vi "Ex 06-5 - Multiple Channels B-Scan With Logging.vi"() -> ()   [LabVIEW 2015]
uses:
  <instrlib>/MicroPulse/Public/Data/Datatypes/MP - data formatting.ctl
  <instrlib>/MicroPulse/Public/Data/Datatypes/MP - amplitude reporting mode.ctl
  <instrlib>/MicroPulse/Public/Data/Datatypes/MP - averaging.ctl
  <instrlib>/MicroPulse/Public/Data/Datatypes/MP - transmit parameters.ctl
  <instrlib>/MicroPulse/Public/Data/Datatypes/MP - pulser voltage.ctl
  <instrlib>/MicroPulse/Public/Data/Datatypes/MP - pulse damping.ctl
  <instrlib>/MicroPulse/Public/Data/Datatypes/MP - test parameters.ctl
  <instrlib>/MicroPulse/Public/Data/Datatypes/MP - receive parameters.ctl
  <instrlib>/MicroPulse/Public/Data/Datatypes/MP - display gate.ctl
  <instrlib>/MicroPulse/Public/Data/Datatypes/MP - waveform type.ctl
  <instrlib>/MicroPulse/Public/Data/Datatypes/MP - analogue filter.ctl
  <instrlib>/MicroPulse/Public/Data/Datatypes/MP - frequency filter.ctl
  <instrlib>/MicroPulse/Public/Data/Datatypes/MP - digital filtering.ctl
  <instrlib>/MicroPulse/Public/Data/Datatypes/MP - high pass filter.ctl
  <instrlib>/MicroPulse/Public/Data/Datatypes/MP - low pass filter.ctl
  <instrlib>/MicroPulse/Public/Data/Datatypes/TCP config.ctl
  <instrlib>/MicroPulse/Public/Data/Datatypes/MP - data output format.ctl
  <instrlib>/MicroPulse/Public/Data/Datatypes/MP - sample frequency.ctl
  <instrlib>/MicroPulse/Public/Data/Datatypes/MP - instrument type.ctl
  <instrlib>/MicroPulse/Public/Data/Datatypes/MP - fly scan range (timed).ctl
  <instrlib>/MicroPulse/Public/Data/Datatypes/MP - inspection direction.ctl
  <instrlib>/MicroPulse/Public/Data/Datatypes/PNDT - colour map selector.ctl
  <instrlib>/MicroPulse/Examples/SubVIs/Main Program State - Enum.ctl
  <instrlib>/MicroPulse/Public/Helper VIs/Low Level/FGV - B-Scan Active - Action [Enum].ctl
  <vilib>/ErrorRing/Error Ring.xnode
  <instrlib>/MicroPulse/MicroPulse_Driver.lvlib
panel:
  in  "Colour Map":T1
  out "B-Scan In Progress?":bool
  in  "Stop Scan":bool
  out "live error out":errorcluster
  out "live error out 2":errorcluster
  in  "Centre Cursor 2":bool
  out "B-Scan Chart 2":u16[][](graph)
  in  "Centre Cursor":bool
  out "B-Scan Chart":u16[][](graph)
  out "Instrument Type":T2
  out "Sample Frequency out":T3 caption="Sample Frequency"
  out "Stop":bool
  in  "Sample Frequency":T3
  in  "PRF":u16=20000 caption="[PRF]" min=1 max=20000 step=100 format="%dHz"
  in  "Data Output Format":T4=enum."8-bit Mode" caption="[DOF]"
  out "A-Scan + Peaks 2":cluster{"timebase":dbl[], "data":u16[]}[](graph) caption="A-Scan + Peaks Test 2"
  out "running average PRF 2":dbl format="%0.2f"
  in  "Channel Tab":enum32{"Test 1", "Test 2", "Inspection"}(tab)
  in  "Test 1 Tab":enum32{"Ultrasonic Parameters"}(tab)
  in  "Data Formatting":T5={"Amplitude Mode"=enum."Peaks + Ascan for Multigate", "Averaging"=enum."None", "Coupling Level"=0} {"Coupling Level" max=4095 step=1}
  in  "Transmit Parameters":T8={"Pulse Voltage"=enum."50V", "Pulse Shape"={"Damping"=enum."660W", "Width"=250}} {"Pulse Shape"."Width" min=16 max=1010 step=50 format="%.0fns"}
  in  "Test Parameters":T11={"Test No."=1, "Tx Channel"=1, "Rx Channel"=1} {"Rx Channel" min=1 max=1024; "Tx Channel" min=1 max=1024}
  in  "Receive Parameters":T12={"Display Gate"={"Start"=0.0, "Length"=100.0}, "Delay"=0.0, "Waveform Type"=enum."Rectified Signal", "Gain"=50.0, "Analogue Filtering"={"Bandpass"=enum."No change", "Smoothing"=1}, "Digital Filtering"={"High Pass Filter"=enum."None", "Low Pass Filter"=enum."None"}} {"Delay" format="%#_g us"; "Display Gate"."Length" min=0.0 max=64000.0 step=1.0 format="%#_g us"; "Display Gate"."Start" min=0.0 max=64000.0 step=1.0 format="%#_g us"; "Analogue Filtering"."Smoothing" min=1 max=11 step=1; "Gain" min=-6.0 max=70.0 step=0.25 format="%.2fdB"}
  in  "Test 1 Tab 2":enum32{"Ultrasonic Parameters"}(tab)
  in  "Data Formatting 2":T5={"Amplitude Mode"=enum."Peaks + Ascan for Multigate", "Averaging"=enum."None", "Coupling Level"=0} {"Coupling Level" max=4095 step=1}
  in  "Transmit Parameters 2":T8={"Pulse Voltage"=enum."50V", "Pulse Shape"={"Damping"=enum."660W", "Width"=250}} {"Pulse Shape"."Width" min=16 max=1010 step=50 format="%.0fns"}
  in  "Test Parameters 2":T11={"Test No."=1, "Tx Channel"=2, "Rx Channel"=2} {"Rx Channel" min=1 max=1024; "Tx Channel" min=1 max=1024}
  in  "Receive Parameters 2":T12={"Display Gate"={"Start"=0.0, "Length"=100.0}, "Delay"=0.0, "Waveform Type"=enum."Rectified Signal", "Gain"=50.0, "Analogue Filtering"={"Bandpass"=enum."No change", "Smoothing"=1}, "Digital Filtering"={"High Pass Filter"=enum."None", "Low Pass Filter"=enum."None"}} {"Delay" format="%#_g us"; "Display Gate"."Length" min=0.0 max=64000.0 step=1.0 format="%#_g us"; "Display Gate"."Start" min=0.0 max=64000.0 step=1.0 format="%#_g us"; "Analogue Filtering"."Smoothing" min=1 max=11 step=1; "Gain" min=-6.0 max=70.0 step=0.25 format="%.2fdB"}
  in  "Log Data?":bool caption="Log Data At End Of Scan?"
  out "Scan Timer Enabled?":bool
  in  "Start Timed Test":bool
  in  "Timed Scan definition":T20={"Max Scan Length"=1200, "Update Rate"=500, "Direction"=enum."Forwards"} {"Update Rate" format="%#_6f"; "Max Scan Length" format="%#_6f"}
  out "A-Scan + Peaks":cluster{"timebase":dbl[], "data":u16[]}[](graph) caption="A-Scan + Peaks Test 1"
  in  "Single Scan":bool
  in  "Stop Streaming":bool
  in  "Start Streaming":bool
  out "Command List":string
  in  "QUIT":bool
  out "running average PRF":dbl format="%0.2f"
  out "System Messages":string
  in  "TCP config":T22={"Connection ID"=refnum, "IP address"="10.1.1.2", "host port"=1067, "OC timeout"=5000, "Read timeout"=2000, "Write timeout"=100} {"Write timeout" format="%dms"; "Read timeout" format="%dms"; "OC timeout" format="%dms"}
  # "Example 06-5 - Multiple Channels B-Scan\n\nSet all controls to the required values\nbefore running the VI."
  # "Tx and Rx Channels MUST be set BEFORE running"
  # "TEST 1"
  # "TEST 2"
  # "Set to zero for unlimited points. Requires manual stop."
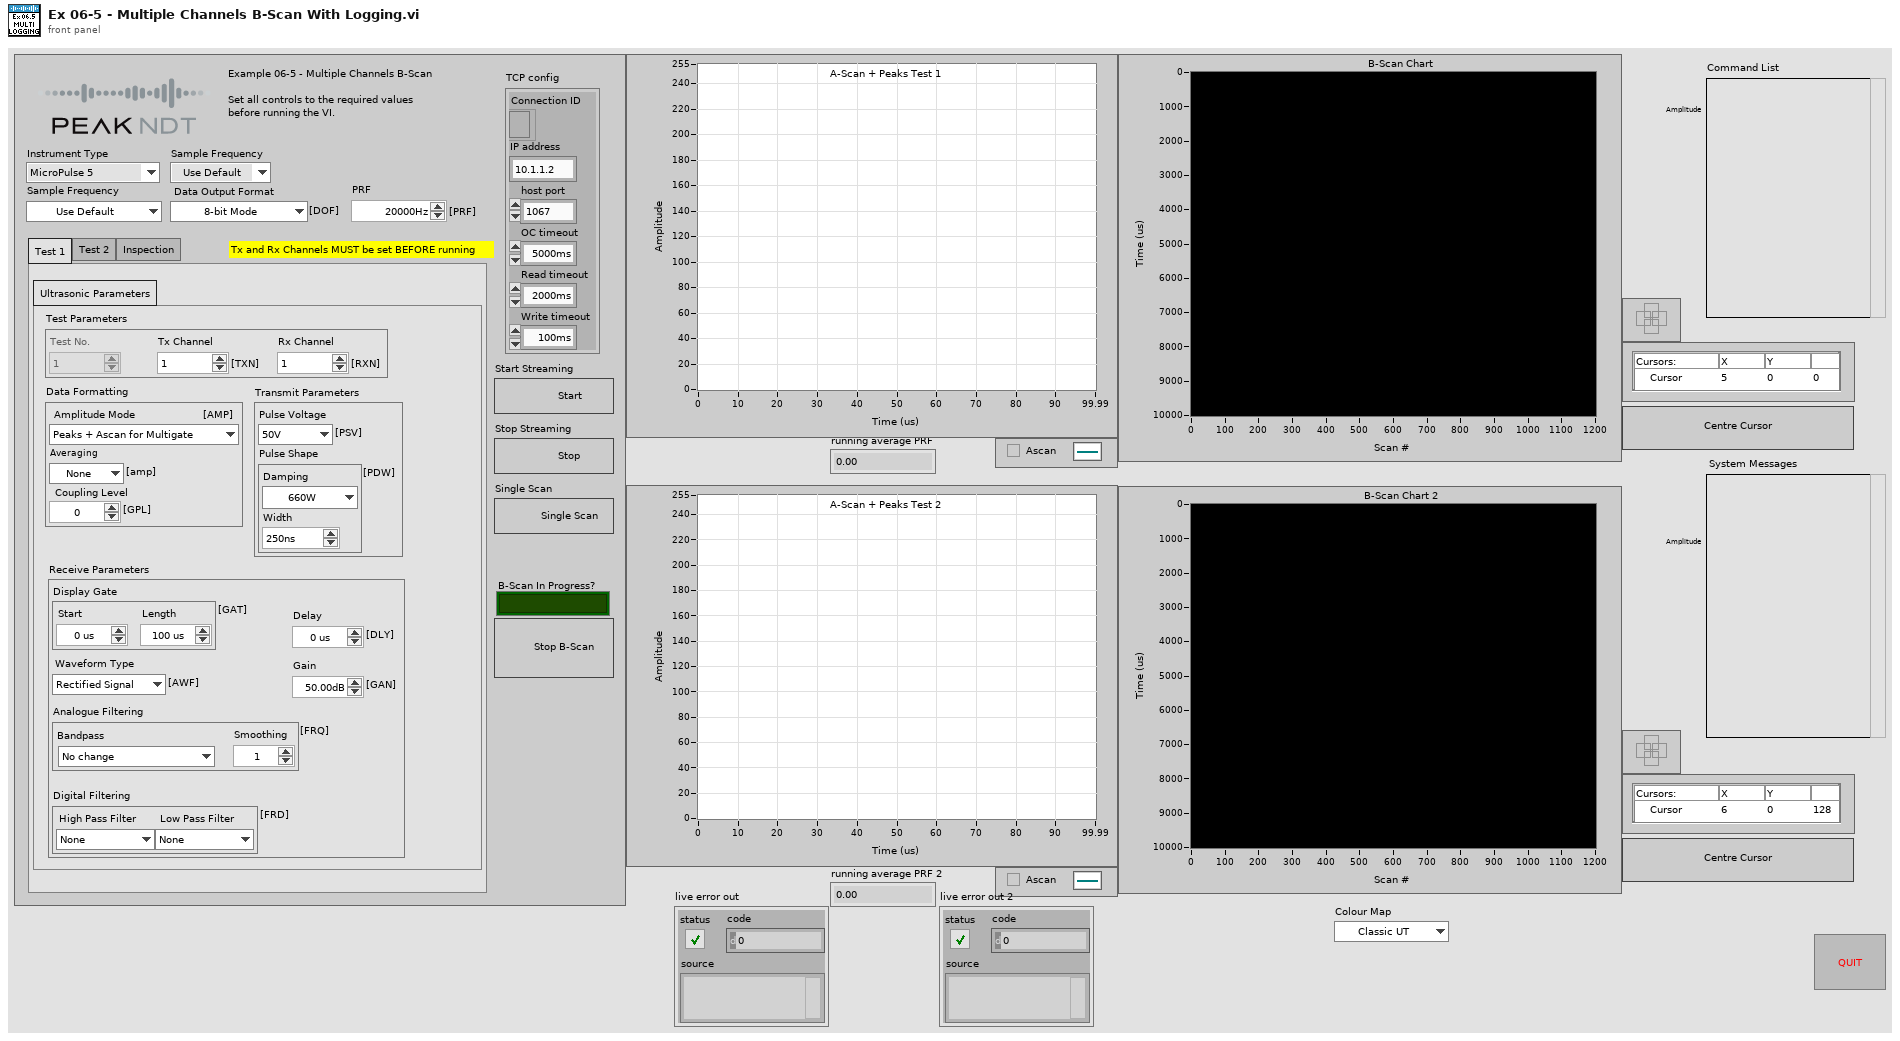
[diagram p1: front panel]
types:
  T1 = typedef "MicroPulse_Driver.lvlib/PNDT - colour map selector.ctl" = enum16{"Classic UT", "Ultrasonic", "Inverse Grey", "Grey Scale", "TOFD", "Fire", "Rainbow", "Ice", "Original"}
  T2 = typedef "MicroPulse_Driver.lvlib/MP - instrument type.ctl" = enum16{"MicroPulse 5", "LT1", "LT2", "LTPA", "MPLT", "MicroPulse 6", "PipeScanner", "<MicroPulse>", "Micropulse 4", "Simulated Data"}
  T3 = typedef "MicroPulse_Driver.lvlib/MP - sample frequency.ctl" = enum16{"Use Default", "200MHz (LT2 only)", "100MHz", "50MHz", "25MHz", "10MHz"}
  T4 = typedef "MicroPulse_Driver.lvlib/MP - data output format.ctl" = enum16{"", "8-bit Mode", "10-bit Mode", "12-bit Mode", "16-bit Mode", "8-bit Log Mode", "12-bit Packed Mode"}
  T5 = typedef "MicroPulse_Driver.lvlib/MP - data formatting.ctl" = cluster{"Amplitude Mode":T6, "Averaging":T7, "Coupling Level":u32}
  T6 = typedef "MicroPulse_Driver.lvlib/MP - amplitude reporting mode.ctl" = enum16{"1st Peak in gate", "Maximum Peak in gate", "All Peaks", "Ascan Data", "1st Threshold Crossing Peak", "Ascan + Peaks", "All Peaks for Multigate", "Peaks + Ascan for Multigate", "Peaks + P_Ascan for Multigate", "Full Matrix Capture"}
  T7 = typedef "MicroPulse_Driver.lvlib/MP - averaging.ctl" = enum16{"None", "2", "4", "8", "16", "32", "64", "128", "256"}
  T8 = typedef "MicroPulse_Driver.lvlib/MP - transmit parameters.ctl" = cluster{"Pulse Voltage":T9, "Pulse Shape":cluster{"Damping":T10, "Width":u32}}
  T9 = typedef "MicroPulse_Driver.lvlib/MP - pulser voltage.ctl" = enum16{"50V", "100V", "150V", "200V", "250V", "300V"}
  T10 = typedef "MicroPulse_Driver.lvlib/MP - pulse damping.ctl" = enum16{"660W", "458W", "220W", "149W", "102W", "82W", "63W", "51W"}
  T11 = typedef "MicroPulse_Driver.lvlib/MP - test parameters.ctl" = cluster{"Test No.":u32, "Tx Channel":u32, "Rx Channel":u32}
  T12 = typedef "MicroPulse_Driver.lvlib/MP - receive parameters.ctl" = cluster{"Display Gate":T13, "Delay":dbl, "Waveform Type":T14, "Gain":dbl, "Analogue Filtering":T15, "Digital Filtering":T17}
  T13 = typedef "MicroPulse_Driver.lvlib/MP - display gate.ctl" = cluster{"Start":dbl, "Length":dbl}
  T14 = typedef "MicroPulse_Driver.lvlib/MP - waveform type.ctl" = enum16{"Rectified Signal", "RF Signal", "+Half Wave", "-Half Wave"}
  T15 = typedef "MicroPulse_Driver.lvlib/MP - analogue filter.ctl" = cluster{"Bandpass":T16, "Smoothing":u16}
  T16 = typedef "MicroPulse_Driver.lvlib/MP - frequency filter.ctl" = enum16{"No change", "1MHz Bandpass", "2MHz Bandpass", "4MHz Bandpass", "5MHz Bandpass", "10MHz Bandpass", "2.5-18MHz Broadband", "0.75-12MHz  Broadband", "0.5MHz Bandpass", "5MHz 2nd Order TOFD", "10MHz 2nd Order TOFD", "3.0-25MHz Broadband", "3.0-30MHz Broadband"}
  T17 = typedef "MicroPulse_Driver.lvlib/MP - digital filtering.ctl" = cluster{"High Pass Filter":T18, "Low Pass Filter":T19}
  T18 = typedef "MicroPulse_Driver.lvlib/MP - high pass filter.ctl" = enum16{"None", "0.7MHz", "1.5MHz", "4.0MHz", "7.5MHz", "10.0MHz", "User Defined"}
  T19 = typedef "MicroPulse_Driver.lvlib/MP - low pass filter.ctl" = enum16{"None", "1.8MHz", "3.0MHz", "6.0MHz", "8.0MHz", "12.0MHz", "User Defined"}
  T20 = typedef "MicroPulse_Driver.lvlib/MP - fly scan range (timed).ctl" = cluster{"Max Scan Length":i32, "Update Rate":i32, "Direction":T21}
  T21 = typedef "MicroPulse_Driver.lvlib/MP - inspection direction.ctl" = enum16{"Forwards", "Backwards"}
  T22 = typedef "MicroPulse_Driver.lvlib/TCP config.ctl" = cluster{"Connection ID":refnum<k5>, "IP address":string, "host port":u16, "OC timeout":i32, "Read timeout":i32, "Write timeout":i32}
  T23 = typedef "Main Program State - Enum.ctl" = enum16{"Initialise", "Init HW", "Run", "Reset HW", "Shutdown"}
  T24 = typedef "MicroPulse_Driver.lvlib/FGV - B-Scan Active - Action [Enum].ctl" = enum16{"Read", "Read & Reset Start Flag", "Start B-Scan", "B-Scan Finished"}
  T25 = typedef "MicroPulse_Driver.lvlib/MP-Registry Data-Cluster.ctl" = cluster{"Instrument Type":T2, "Serial #":u64, "Sample Frequency":T3, "dt (us)":dbl, "DOF":T4, "Material Velocity":dbl, "Asynch Reads":T26, "NUM of Tests":u32, "System Details":T27, "Gates":T29[], "Encoders":T35[], "CMD LUT":variant, "Command List":string}
  T26 = typedef "MicroPulse_Driver.lvlib/MP - asynch read mode.ctl" = enum16{"Disabled", "Enabled"}
  T27 = typedef "MicroPulse_Driver.lvlib/MP - general system status.ctl" = cluster{"System Type":T2, "Serial No.":u64, "Channels":cluster{"Conv":u8, "PA":u16, "Extra":u32}, "Sample Frequency":cluster{"Default":u8, "Actual":u8}, "Software Versions":string, "Data Output Format":cluster{"Default":T4, "Actual":T4}, "Temperatures":cluster{"System":u8, "Processor":u8, "Slave Sys":u8, "Slave Proc":u8}, "Tx Buffer Size":u32, "System Error":string, "No. of Cards":u8, "DAC Gain":i16, "Uptimes":cluster{"since Power":u32, "since RSTS":u32, "since SRST":u32}, "Voltages":cluster{"Nominal":dbl, "Measured":dbl, "Difference":dbl}[], "Interface Cards":T28[]}
  T28 = typedef "MicroPulse_Driver.lvlib/MP - interface card status.ctl" = cluster{"Status":u8, "Map":u8, "Board - T":u8, "FPGA - T":u8, "PAIF Status":string, "Version":string}
  T29 = typedef "MicroPulse_Driver.lvlib/MP - Registry Gates.ctl" = cluster{"Display Gate":T13, "ETM Mode":T30, "Echo Gate":T31, "Insp Gates":T32[]}
  T30 = typedef "MicroPulse_Driver.lvlib/MP - echo gate mode.ctl" = enum16{"Echo Trigger OFF", "Echo Gate Display Mode", "Echo Trigger ON", "Multi Gate or FMC Mode", "Reserved", "PA - Echo Trigger ON"}
  T31 = typedef "MicroPulse_Driver.lvlib/MP - echo gate parameters.ctl" = cluster{"Start (us)":dbl, "Length (us)":dbl, "Threshold":u16, "Colour":u32}
  T32 = typedef "MicroPulse_Driver.lvlib/MP - multigate inspection gate parameters.ctl" = cluster{"Start (us)":dbl, "Length (us)":dbl, "Threshold":u16, "Enabled?":bool, "Max # Peaks":u16, "Hysteresis":T33, "Mode":T34, "Inverted?":bool, "Colour ":u32}
  T33 = typedef "MicroPulse_Driver.lvlib/MP - hysteresis level.ctl" = enum16{"None", "3dB", "6dB", "9dB", "12dB"}
  T34 = typedef "MicroPulse_Driver.lvlib/MP - multigate mode.ctl" = enum16{"1st Peak in Gate", "Largest Peak In Gate", "All Peaks In Gate", "1st Threshold Crossing"}
  T35 = typedef "MicroPulse_Driver.lvlib/MP - encoder settings.ctl" = cluster{"Encoder Type":T36, "Counts/mm":u32, "Enable Termination?":bool, "Multiplier":u32, "Backlash Period (s)":dbl, "Encoder Filter":u32}
  T36 = typedef "MicroPulse_Driver.lvlib/MP - encoder type.ctl" = enum16{"Quadrature", "Step/Direction"}
  T37 = typedef "MicroPulse_Driver.lvlib/MP - scan data info.ctl" = cluster{"Message Header":u16, "Error Message":u16, "Test No.":u32, "Channel No.":u8, "Sweep No.":u32, "Gate No.":u32, "DOF":T4, "retain data":T38, "scan data":u16[], "scan length":i32, "scan index":i32, "peak data":cluster{"timebase":u16[], "data":u16[]}, "#peaks":i32, "PRF":dbl, "IP":cluster{"Axis No.":u8, "Location":u32, "MIP location":u32, "MIP?":bool}, "echo range":u16, "ETG":bool, "CAL 0 complete":bool, "Axis Positions":T39}
  T38 = typedef "MicroPulse_Driver.lvlib/MP - retain scan.ctl" = enum16{"None", "Ascan", "Peaks"}
  T39 = typedef "MicroPulse_Driver.lvlib/MP - axis positions (LLC).ctl" = cluster{"Axis 1":u32, "Axis 2":u32, "Axis 3":u32, "Axis 4":u32, "Status":u8}
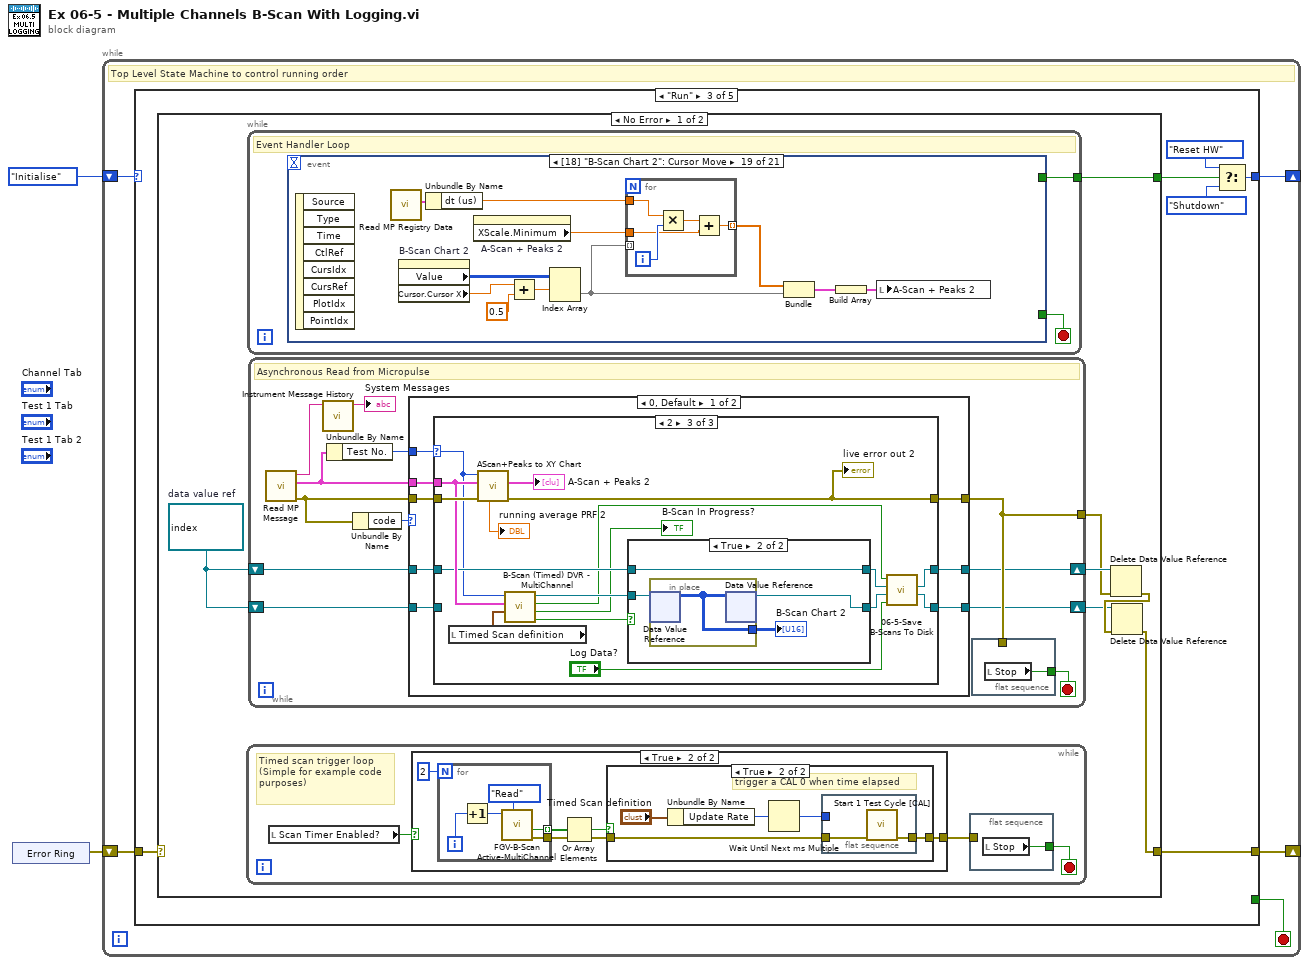
[diagram p0: block diagram]
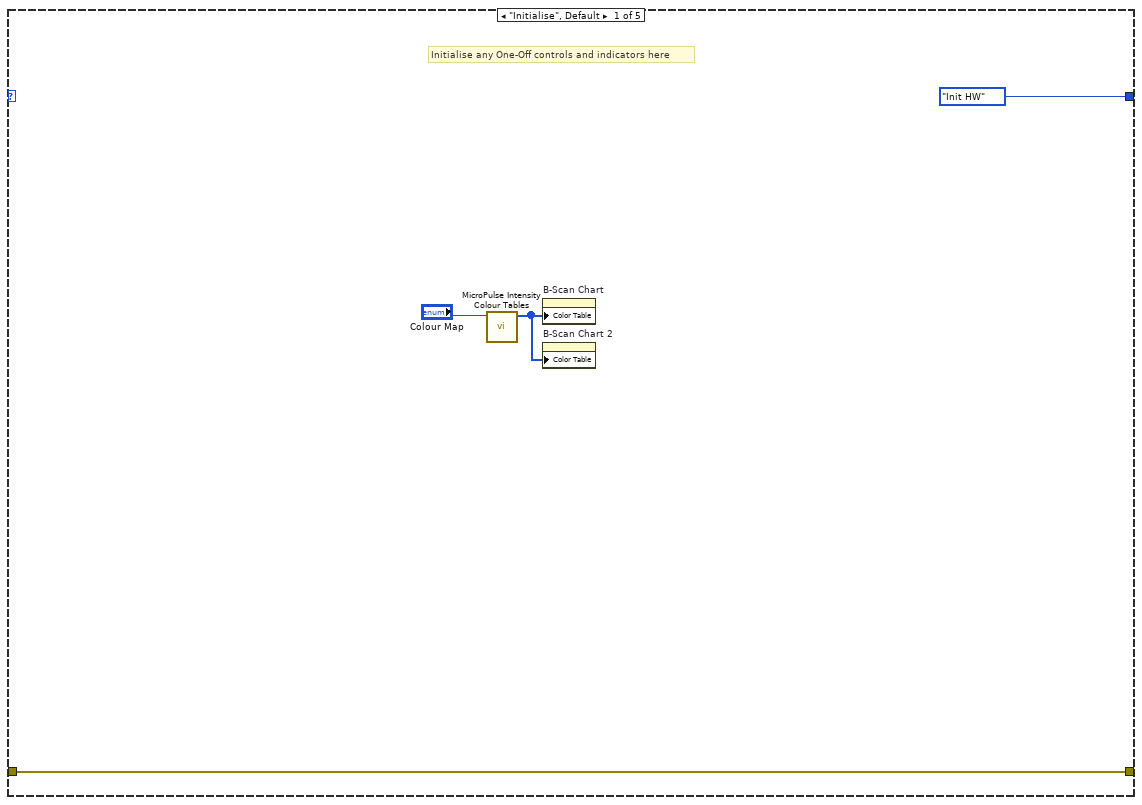
[diagram p2: hidden frame]
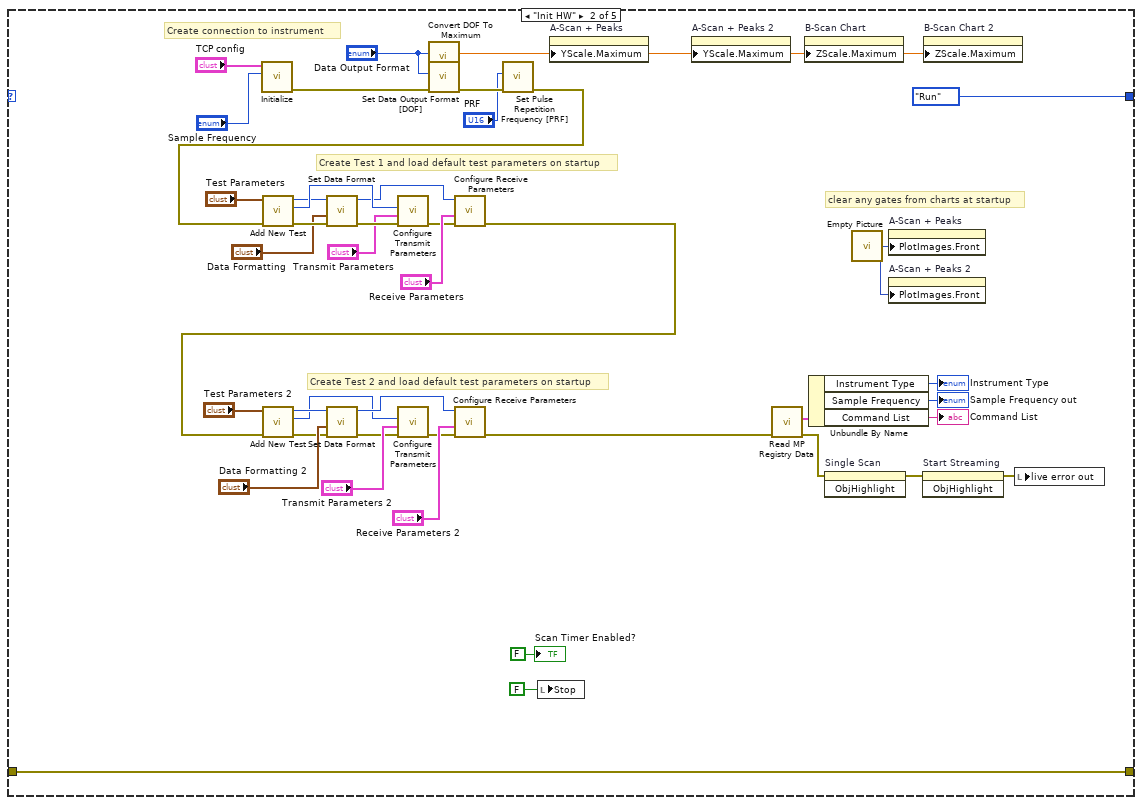
[diagram p3: hidden frame]
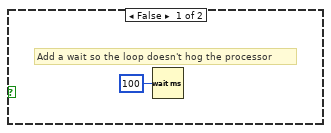
[diagram p4: hidden frame]
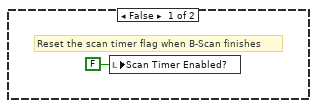
[diagram p5: hidden frame]
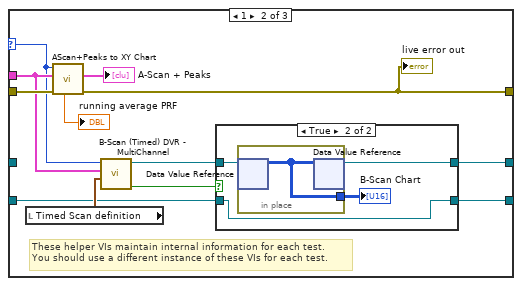
[diagram p7: hidden frame]
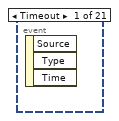
[diagram p11: hidden frame]
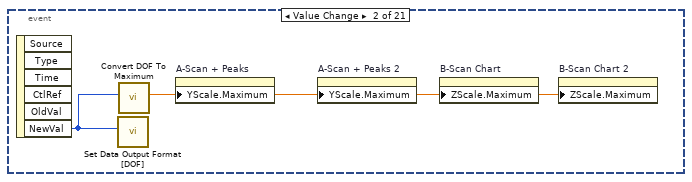
[diagram p12: hidden frame]
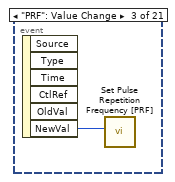
[diagram p13: hidden frame]
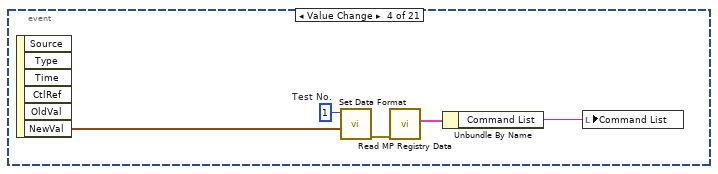
[diagram p14: hidden frame]
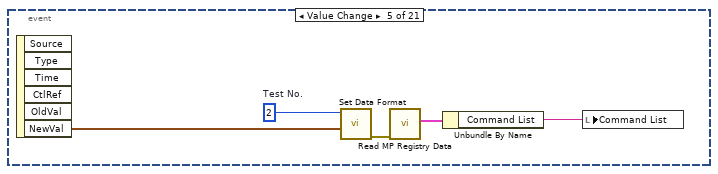
[diagram p15: hidden frame]
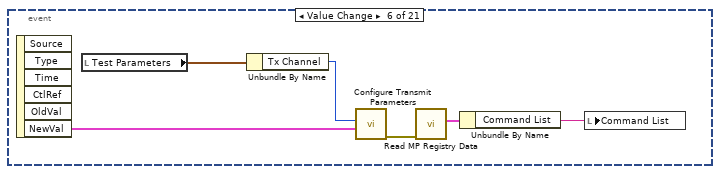
[diagram p16: hidden frame]
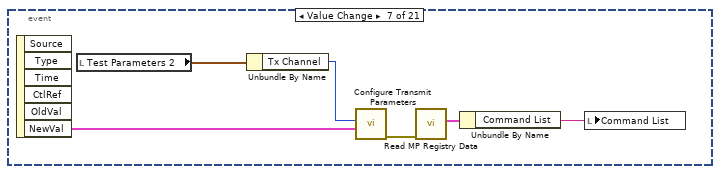
[diagram p17: hidden frame]
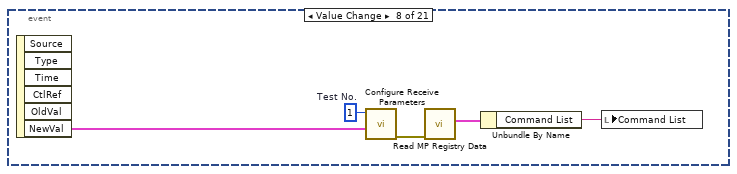
[diagram p18: hidden frame]
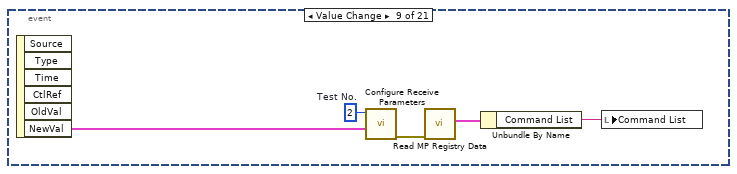
[diagram p19: hidden frame]
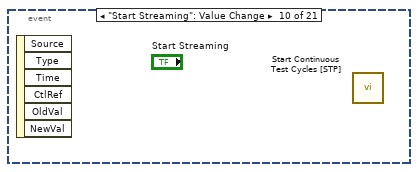
[diagram p20: hidden frame]
diagram:
  n1 = xnode "Error Ring"() -> ("error out"=w2:errorcluster)
  n2 = while {
    shift-right: [w4] -> _
    shift-left: Main_Program_State_-_Enum."Initialise" -> [w7]
    shift-right: [w5] -> _
    shift-left: w2 -> [w6]
    stop <- w3 stop-if-true
    # "Top Level State Machine to control running order"
    n3 = case shown="\"Run\"" w7 {
      tunnel: w6 -> [w10 w28 w59 w276 w281]
      tunnel: [w10 w28 w58 w275 w281] -> w5
      tunnel: [Main_Program_State_-_Enum."Init HW" Main_Program_State_-_Enum."Run" w54 Main_Program_State_-_Enum."Init HW" Main_Program_State_-_Enum."Initialise"] -> w4
      tunnel: [_ _ _ _ TRUE] -> w3
      frame "Initialise", Default {
        # "Initialise any One-Off controls and indicators here"
        n4 = call <instrlib>:"MicroPulse Intensity Colour Tables.vi"("Colour Map Type"="Colour Map") -> ("Colour Table"=w8:u32[])  [unwired: 10 in]
        n5 = property on="B-Scan Chart" class="IntGraph (strict)"("Color Table"=w8) -> ()  [unwired: 2 in, 2 out]
        n6 = property on="B-Scan Chart 2" class="IntGraph (strict)"("Color Table"=w8) -> ()  [unwired: 2 in, 2 out]
      }
      frame "Init HW" {
        # "Create connection to instrument"
        # "Create Test 2 and load default test parameters on startup"
        # "clear any gates from charts at startup"
        # "Create Test 1 and load default test parameters on startup"
        n7 = call <instrlib>:"Initialize.vi"("Sample Frequency"="Sample Frequency", "TCP config"="TCP config") -> ("error out"=w21:errorcluster)  [unwired: 8 in, 1 out]
        n8 = call <instrlib>:"Convert DOF To Maximum.vi"("Data Output Format"="Data Output Format") -> ("Data Maximum"=w12:dbl)  [unwired: 10 in]
        n9 = call <instrlib>:"Set Data Output Format [DOF].vi"("error in (no error)"=w21, "Mode"="Data Output Format") -> ("error out"=w23:errorcluster)  [unwired: 8 in, 1 out]
        n10 = call <instrlib>:"Set Pulse Repetition Frequency [PRF].vi"("error in (no error)"=w23, "Frequency (Hz)"="PRF") -> ("error out"=w20:errorcluster)  [unwired: 8 in, 1 out]
        n11 = call <instrlib>:"Add New Test.vi"("error in (no error)"=w20, "Test Parameters"="Test Parameters") -> ("error out"=w39:errorcluster, "Tx Channel out"=w38:u32, "Test No. out"=w36:u32)  [unwired: 6 in, 1 out]
        n12 = call <instrlib>:"Set Data Format.vi"("error in (no error)"=w39, "Data Formatting"="Data Formatting", "Test No."=w36) -> ("error out"=w33:errorcluster, "Test No. out"=w37:u32)  [unwired: 6 in, 1 out]
        n13 = call <instrlib>:"Configure Transmit Parameters.vi"("error in (no error)"=w33, "Transmit Parameters"="Transmit Parameters", "Tx Channel"=w38) -> ("error out"=w32:errorcluster)  [unwired: 7 in, 1 out]
        n14 = call <instrlib>:"Configure Receive Parameters.vi"("error in (no error)"=w32, "Receive Parameters"="Receive Parameters", "Test No."=w37) -> ("error out"=w16:errorcluster)  [unwired: 6 in, 2 out]
        n15 = call <instrlib>:"Add New Test.vi"("error in (no error)"=w16, "Test Parameters"="Test Parameters 2") -> ("error out"=w48:errorcluster, "Tx Channel out"=w44:u32, "Test No. out"=w46:u32)  [unwired: 6 in, 1 out]
        n16 = call <instrlib>:"Set Data Format.vi"("error in (no error)"=w48, "Data Formatting"="Data Formatting 2", "Test No."=w46) -> ("error out"=w49:errorcluster, "Test No. out"=w45:u32)  [unwired: 6 in, 1 out]
        n17 = call <instrlib>:"Configure Transmit Parameters.vi"("error in (no error)"=w49, "Transmit Parameters"="Transmit Parameters 2", "Tx Channel"=w44) -> ("error out"=w50:errorcluster)  [unwired: 7 in, 1 out]
        n18 = call <instrlib>:"Configure Receive Parameters.vi"("error in (no error)"=w50, "Receive Parameters"="Receive Parameters 2", "Test No."=w45) -> ("error out"=w15:errorcluster)  [unwired: 6 in, 2 out]
        n19 = local write "Stop"(FALSE ("stop")) -> ()
        n20 = property on="A-Scan + Peaks" class="XYGraph (strict)"("YScale.Maximum"=w12) -> ()  [unwired: 2 in, 2 out]
        n21 = property on="A-Scan + Peaks 2" class="XYGraph (strict)"("YScale.Maximum"=w12) -> ()  [unwired: 2 in, 2 out]
        n22 = call <instrlib>:"Read MP Registry Data.vi"("error in (no error)"=w15) -> ("error out"=w42:errorcluster, "Micropulse Data"=w40:T25)  [unwired: 7 in, 2 out]
        n23 = property on="B-Scan Chart" class="IntGraph (strict)"("ZScale.Maximum"=w12) -> ()  [unwired: 2 in, 2 out]
        n24 = Unbundle By Name(w40) -> ("Instrument Type"=→"Instrument Type":T2, "Sample Frequency"=→"Sample Frequency out":T3, "Command List"=→"Command List":string)
        n25 = invoke on="Single Scan" class="Bool" method="ObjHighlight"(error in=w42) -> (error out=w43:errorcluster)  [unwired: 2 in, 2 out]
        n26 = call "Empty Picture"() -> ("empty picture"=w27:picture)
        n27 = property on="A-Scan + Peaks" class="XYGraph (strict)"("PlotImages.Front"=w27) -> ()  [unwired: 2 in, 2 out]
        n28 = property on="A-Scan + Peaks 2" class="XYGraph (strict)"("PlotImages.Front"=w27) -> ()  [unwired: 2 in, 2 out]
        n29 = invoke on="Start Streaming" class="Bool" method="ObjHighlight"(error in=w43) -> (error out=w13:errorcluster)  [unwired: 2 in, 2 out]
        n30 = property on="B-Scan Chart 2" class="IntGraph (strict)"("ZScale.Maximum"=w12) -> ()  [unwired: 2 in, 2 out]
        n31 = local write "live error out"(w13) -> ()
        "Scan Timer Enabled?" <- FALSE ("Scan Timer Enabled?")
      }
      frame "Run" {
        n32 = case shown="No Error" w59 {
          selector: w59 -> [_ w274]
          tunnel: [w61 w274] -> w58
          tunnel: [w66 _] -> w55
          frame No Error {
            w65 = refnum<data-value> refnum  # data value ref
            n33 = while {
              stop <- w68 stop-if-true
              # "Timed scan trigger loop\n(Simple for example code purposes)"
              n34 = local read "Scan Timer Enabled?"() -> (w69:bool)
              n35 = case shown="True" w69 {
                tunnel: [_ w72] -> w67
                frame False {
                  # "Add a wait so the loop doesn't hog the processor"
                  n36 = Wait (ms)(milliseconds to wait=u32 100) -> ()  [unwired: 1 out]
                }
                frame True {
                  n37 = for {
                    N: 2 -> [_]
                    tunnel: [w80] -> w76 mode=indexing
                    tunnel: [w79] -> w75
                    i -> [w77]
                    n38 = Increment(x=w77) -> (x+1=w78:i32)
                    n39 = call <instrlib>:"FGV-B-Scan Active-MultiChannel.vi"("Action"=FGV_-_B-Scan_Active_-_Action_[Enum]."Read", "Test #"=w78) -> ("error out"=w79:errorcluster, "B-Scan In Progress?"=w80:bool)  [unwired: 7 in, 1 out]
                  }
                  n40 = Or Array Elements(Boolean array=w76) -> (logical OR=w73:bool)
                  n41 = case shown="True" w73 {
                    tunnel: w75 -> [_ w85]
                    tunnel: [_ w83] -> w72
                    frame False {
                      # "Reset the scan timer flag when B-Scan finishes"
                      n42 = local write "Scan Timer Enabled?"(FALSE ("Scan Timer Enabled?")) -> ()
                    }
                    frame True {
                      # "trigger a CAL 0 when time elapsed"
                      n43 = Unbundle By Name("Timed Scan definition") -> ("Update Rate"=w87:i32)
                      n44 = Wait Until Next ms Multiple(millisecond multiple=w87) -> (millisecond timer value=w86:u32)
                      n45 = flat-sequence {
                        tunnel: w86 -> [_]
                        tunnel: w85 -> [w89]
                        tunnel: [w88] -> w83
                        frame #0 {
                          n46 = call <instrlib>:"Start 1 Test Cycle [CAL].vi"("error in (no error)"=w89) -> ("error out"=w88:errorcluster)  [unwired: 9 in, 1 out]
                        }
                      }
                    }
                  }
                }
              }
              n47 = flat-sequence {
                tunnel: [w70] -> w68
                tunnel: w67 -> [_]
                frame #0 {
                  n48 = local read "Stop"() -> (w70:bool)
                }
              }
            }
            n49 = while {
              tunnel: [w160] -> w66
              stop <- w161 stop-if-true
              # "Event Handler Loop"
              n50 = event shown="[18] \"B-Scan Chart 2\": Cursor Move" {
                selector: _ -> [_ _ _ _ _ _ _ _ _ _ _ _ _ _ _ _ _ _ _ _ _]
                dyn-events: _ -> [_ _ _ _ _ _ _ _ _ _ _ _ _ _ _ _ _ _ _ _ _]
                timeout: _ -> [_ _ _ _ _ _ _ _ _ _ _ _ _ _ _ _ _ _ _ _ _]
                tunnel: [_ _ _ _ _ _ _ _ _ _ _ _ w198 _ _ _ _ _ _ _ TRUE ("stop")] -> w161
                tunnel: [_ _ _ _ _ _ _ _ _ _ _ _ TRUE _ _ _ _ _ _ _ _] -> w160
                event Timeout {
                  n51 = event-data() -> ()  [unwired: 1 in, 3 out]
                }
                event Value Change {
                  n52 = event-data() -> ("NewVal"=w163:T4)  [unwired: 1 in, 5 out]
                  n53 = call <instrlib>:"Set Data Output Format [DOF].vi"("Mode"=w163) -> ()  [unwired: 9 in, 2 out]
                  n54 = call <instrlib>:"Convert DOF To Maximum.vi"("Data Output Format"=w163) -> ("Data Maximum"=w162:dbl)  [unwired: 10 in]
                  n55 = property on="A-Scan + Peaks" class="XYGraph (strict)"("YScale.Maximum"=w162) -> ()  [unwired: 2 in, 2 out]
                  n56 = property on="A-Scan + Peaks 2" class="XYGraph (strict)"("YScale.Maximum"=w162) -> ()  [unwired: 2 in, 2 out]
                  n57 = property on="B-Scan Chart" class="IntGraph (strict)"("ZScale.Maximum"=w162) -> ()  [unwired: 2 in, 2 out]
                  n58 = property on="B-Scan Chart 2" class="IntGraph (strict)"("ZScale.Maximum"=w162) -> ()  [unwired: 2 in, 2 out]
                }
                event "PRF": Value Change {
                  n59 = event-data() -> ("NewVal"=w164:u16)  [unwired: 1 in, 5 out]
                  n60 = call <instrlib>:"Set Pulse Repetition Frequency [PRF].vi"("Frequency (Hz)"=w164) -> ()  [unwired: 9 in, 2 out]
                }
                event Value Change {
                  w166 = u32 1  # Test No.
                  n61 = event-data() -> ("NewVal"=w165:T5)  [unwired: 1 in, 5 out]
                  n62 = call <instrlib>:"Set Data Format.vi"("Data Formatting"=w165, "Test No."=w166) -> ("error out"=w169:errorcluster)  [unwired: 7 in, 2 out]
                  n63 = call <instrlib>:"Read MP Registry Data.vi"("error in (no error)"=w169) -> ("Micropulse Data"=w168:T25)  [unwired: 7 in, 3 out]
                  n64 = Unbundle By Name(w168) -> ("Command List"=w167:string)
                  n65 = local write "Command List"(w167) -> ()
                }
                event Value Change {
                  w171 = u32 2  # Test No.
                  n66 = event-data() -> ("NewVal"=w170:T5)  [unwired: 1 in, 5 out]
                  n67 = call <instrlib>:"Set Data Format.vi"("Data Formatting"=w170, "Test No."=w171) -> ("error out"=w174:errorcluster)  [unwired: 7 in, 2 out]
                  n68 = call <instrlib>:"Read MP Registry Data.vi"("error in (no error)"=w174) -> ("Micropulse Data"=w173:T25)  [unwired: 7 in, 3 out]
                  n69 = Unbundle By Name(w173) -> ("Command List"=w172:string)
                  n70 = local write "Command List"(w172) -> ()
                }
                event Value Change {
                  n71 = event-data() -> ("NewVal"=w179:T8)  [unwired: 1 in, 5 out]
                  n72 = local read "Test Parameters"() -> (w180:T11)
                  n73 = Unbundle By Name(w180) -> ("Tx Channel"=w178:u32)
                  n74 = call <instrlib>:"Configure Transmit Parameters.vi"("Transmit Parameters"=w179, "Tx Channel"=w178) -> ("error out"=w176:errorcluster)  [unwired: 8 in, 1 out]
                  n75 = call <instrlib>:"Read MP Registry Data.vi"("error in (no error)"=w176) -> ("Micropulse Data"=w177:T25)  [unwired: 7 in, 3 out]
                  n76 = Unbundle By Name(w177) -> ("Command List"=w175:string)
                  n77 = local write "Command List"(w175) -> ()
                }
                event Value Change {
                  n78 = event-data() -> ("NewVal"=w185:T8)  [unwired: 1 in, 5 out]
                  n79 = local read "Test Parameters 2"() -> (w186:T11)
                  n80 = Unbundle By Name(w186) -> ("Tx Channel"=w184:u32)
                  n81 = call <instrlib>:"Configure Transmit Parameters.vi"("Transmit Parameters"=w185, "Tx Channel"=w184) -> ("error out"=w182:errorcluster)  [unwired: 8 in, 1 out]
                  n82 = call <instrlib>:"Read MP Registry Data.vi"("error in (no error)"=w182) -> ("Micropulse Data"=w183:T25)  [unwired: 7 in, 3 out]
                  n83 = Unbundle By Name(w183) -> ("Command List"=w181:string)
                  n84 = local write "Command List"(w181) -> ()
                }
                event Value Change {
                  w187 = u32 1  # Test No.
                  n85 = event-data() -> ("NewVal"=w191:T12)  [unwired: 1 in, 5 out]
                  n86 = call <instrlib>:"Configure Receive Parameters.vi"("Receive Parameters"=w191, "Test No."=w187) -> ("error out"=w190:errorcluster)  [unwired: 7 in, 2 out]
                  n87 = call <instrlib>:"Read MP Registry Data.vi"("error in (no error)"=w190) -> ("Micropulse Data"=w188:T25)  [unwired: 7 in, 3 out]
                  n88 = Unbundle By Name(w188) -> ("Command List"=w189:string)
                  n89 = local write "Command List"(w189) -> ()
                }
                event Value Change {
                  w192 = u32 2  # Test No.
                  n90 = event-data() -> ("NewVal"=w196:T12)  [unwired: 1 in, 5 out]
                  n91 = call <instrlib>:"Configure Receive Parameters.vi"("Receive Parameters"=w196, "Test No."=w192) -> ("error out"=w195:errorcluster)  [unwired: 7 in, 2 out]
                  n92 = call <instrlib>:"Read MP Registry Data.vi"("error in (no error)"=w195) -> ("Micropulse Data"=w193:T25)  [unwired: 7 in, 3 out]
                  n93 = Unbundle By Name(w193) -> ("Command List"=w194:string)
                  n94 = local write "Command List"(w194) -> ()
                }
                event "Start Streaming": Value Change {
                  n95 = event-data() -> ()  [unwired: 1 in, 6 out]
                  n96 = call <instrlib>:"Start Continuous Test Cycles [STP].vi"() -> ()  [unwired: 10 in, 2 out]
                }
                event "Stop Streaming": Value Change {
                  w197 = TRUE  # Erase All? (def F)
                  n97 = event-data() -> ()  [unwired: 1 in, 6 out]
                  n98 = call <instrlib>:"Enter Idle Mode [STX].vi"("Erase All? (def T)"=w197) -> ()  [unwired: 9 in, 2 out]
                }
                event "Single Scan": Value Change {
                  n99 = event-data() -> ()  [unwired: 1 in, 6 out]
                  n100 = call <instrlib>:"Start 1 Test Cycle [CAL].vi"() -> ()  [unwired: 10 in, 2 out]
                }
                event Value Change {
                  w198 = TRUE
                  # "Stop all activity and reset the hardware to change the sampling frequency"
                  n101 = event-data() -> ()  [unwired: 1 in, 6 out]
                  n102 = local write "Stop"(w198) -> ()
                }
                event "Start Timed Test": Value Change {
                  # "use property node so we can sequence starting\nthe B-Scan acitve flags and then enabling the timer"
                  # "Stop any acquisition that's going on"
                  n103 = event-data() -> ()  [unwired: 1 in, 6 out]
                  n104 = call <instrlib>:"Enter Idle Mode [STX].vi"() -> ("error out"=w203:errorcluster)  [unwired: 10 in, 1 out]
                  n105 = for {
                    N: 2 -> [_]
                    tunnel: FGV_-_B-Scan_Active_-_Action_[Enum]."Start B-Scan" ("Action") -> [w209]
                    shift-right: [w207] -> w202
                    shift-left: w203 -> [w208]
                    i -> [w205]
                    n106 = Increment(x=w205) -> (x+1=w206:i32)
                    n107 = call <instrlib>:"FGV-B-Scan Active-MultiChannel.vi"("Action"=w209, "error in (no error)"=w208, "Test #"=w206) -> ("error out"=w207:errorcluster)  [unwired: 6 in, 2 out]
                  }
                  n108 = property on="Scan Timer Enabled?" class="Bool (strict)"(error in=w202, "Value"=TRUE ("Scan Timer Enabled?")) -> ()  [unwired: 1 in, 2 out]
                }
                event "Stop Scan": Value Change {
                  n109 = event-data() -> ()  [unwired: 1 in, 6 out]
                  n110 = for {
                    N: 2 -> [_]
                    tunnel: [w216] -> w212 mode=indexing
                    tunnel: [w215] -> _
                    i -> [w213]
                    n111 = Increment(x=w213) -> (x+1=w214:i32)
                    n112 = call <instrlib>:"FGV-B-Scan Active-MultiChannel.vi"("Action"=FGV_-_B-Scan_Active_-_Action_[Enum]."Read", "Test #"=w214) -> ("error out"=w215:errorcluster, "B-Scan In Progress?"=w216:bool)  [unwired: 7 in, 1 out]
                  }
                  n113 = Or Array Elements(Boolean array=w212) -> (logical OR=w210:bool)
                  n114 = case shown="True" w210 {
                    frame False {
                    }
                    frame True {
                      n115 = call <instrlib>:"Enter Idle Mode [STX].vi"("Erase All? (def T)"=FALSE) -> ("error out"=w220:errorcluster)  [unwired: 9 in, 1 out]
                      n116 = for {
                        N: 2 -> [_]
                        tunnel: FGV_-_B-Scan_Active_-_Action_[Enum]."B-Scan Finished" ("Action") -> [w225]
                        tunnel: w220 -> [w224]
                        i -> [w223]
                        n117 = Increment(x=w223) -> (x+1=w222:i32)
                        n118 = call <instrlib>:"FGV-B-Scan Active-MultiChannel.vi"("Action"=w225, "error in (no error)"=w224, "Test #"=w222) -> ()  [unwired: 6 in, 3 out]
                      }
                    }
                  }
                }
                event "Centre Cursor": Value Change {
                  n119 = event-data() -> ()  [unwired: 1 in, 6 out]
                  n120 = property on="B-Scan Chart" class="IntGraph (strict)"() -> ("XScale.Maximum"=w231:dbl, "XScale.Minimum"=w227:dbl)  [unwired: 2 in, 2 out]
                  n121 = Subtract(x=w231, y=w227) -> (x-y=w230:dbl)
                  n122 = Divide(x=w230, y=2.0) -> (x/y=w228:dbl)
                  n123 = Add(x=w228, y=w227) -> (x+y=w226:dbl)
                  n124 = property on="B-Scan Chart" class="IntGraph (strict)"("Cursor.Cursor X"=w226) -> ()  [unwired: 2 in, 2 out]
                }
                event "B-Scan Chart": Cursor Move {
                  n125 = event-data() -> ()  [unwired: 1 in, 8 out]
                  n126 = call <instrlib>:"Read MP Registry Data.vi"() -> ("Micropulse Data"=w236:T25)  [unwired: 8 in, 3 out]
                  n127 = property on="B-Scan Chart" class="IntGraph (strict)"() -> ("Value"=w242:u16[][], "Cursor.Cursor X"=w235:dbl)  [unwired: 2 in, 2 out]
                  n128 = Unbundle By Name(w236) -> ("dt (us)"=w233:dbl)
                  n129 = property on="A-Scan + Peaks" class="XYGraph (strict)"() -> ("XScale.Minimum"=w241:dbl)  [unwired: 2 in, 2 out]
                  n130 = Subtract(x=w235, y=0.5) -> (x-y=w234:dbl)
                  n131 = Index Array(array=w242, index (row)=w234) -> (element=w240:u16[])  [unwired: 1 in]
                  n132 = for {
                    tunnel: w240 -> [_] mode=indexing
                    tunnel: w233 -> [w244]
                    tunnel: w241 -> [w245]
                    tunnel: [w243] -> w239 mode=indexing
                    i -> [w247]
                    n133 = Multiply(x=w244, y=w247) -> (x*y=w246:dbl)
                    n134 = Add(x=w246, y=w245) -> (x+y=w243:dbl)
                  }
                  n135 = Bundle(w239, "Value"=w240) -> (w238:cluster{dbl[], "Value":u16[]})  [unwired: 1 in]
                  n136 = Build Array(w238) -> (w237:cluster{dbl[], "Value":u16[]}[])
                  n137 = local write "A-Scan + Peaks"(w237) -> ()
                }
                event "Centre Cursor 2": Value Change {
                  n138 = event-data() -> ()  [unwired: 1 in, 6 out]
                  n139 = property on="B-Scan Chart 2" class="IntGraph (strict)"() -> ("XScale.Maximum"=w253:dbl, "XScale.Minimum"=w249:dbl)  [unwired: 2 in, 2 out]
                  n140 = Subtract(x=w253, y=w249) -> (x-y=w252:dbl)
                  n141 = Divide(x=w252, y=2.0) -> (x/y=w250:dbl)
                  n142 = Add(x=w250, y=w249) -> (x+y=w248:dbl)
                  n143 = property on="B-Scan Chart 2" class="IntGraph (strict)"("Cursor.Cursor X"=w248) -> ()  [unwired: 2 in, 2 out]
                }
                event "B-Scan Chart 2": Cursor Move {
                  n144 = event-data() -> ()  [unwired: 1 in, 8 out]
                  n145 = call <instrlib>:"Read MP Registry Data.vi"() -> ("Micropulse Data"=w257:T25)  [unwired: 8 in, 3 out]
                  n146 = property on="B-Scan Chart 2" class="IntGraph (strict)"() -> ("Value"=w264:u16[][], "Cursor.Cursor X"=w258:dbl)  [unwired: 2 in, 2 out]
                  n147 = Unbundle By Name(w257) -> ("dt (us)"=w256:dbl)
                  n148 = property on="A-Scan + Peaks 2" class="XYGraph (strict)"() -> ("XScale.Minimum"=w263:dbl)  [unwired: 2 in, 2 out]
                  n149 = Add(x=w258, y=0.5) -> (x+y=w255:dbl)
                  n150 = Index Array(array=w264, index (row)=w255) -> (element=w262:u16[])  [unwired: 1 in]
                  n151 = for {
                    tunnel: w262 -> [_] mode=indexing
                    tunnel: w256 -> [w269]
                    tunnel: w263 -> [w266]
                    tunnel: [w265] -> w261 mode=indexing
                    i -> [w268]
                    n152 = Multiply(x=w269, y=w268) -> (x*y=w267:dbl)
                    n153 = Add(x=w267, y=w266) -> (x+y=w265:dbl)
                  }
                  n154 = Bundle(w261, "Value"=w262) -> (w260:cluster{dbl[], "Value":u16[]})  [unwired: 1 in]
                  n155 = Build Array(w260) -> (w259:cluster{dbl[], "Value":u16[]}[])
                  n156 = local write "A-Scan + Peaks 2"(w259) -> ()
                }
                event Value Change {
                  n157 = event-data() -> ("NewVal"=w270:T1)  [unwired: 1 in, 5 out]
                  n158 = call <instrlib>:"MicroPulse Intensity Colour Tables.vi"("Colour Map Type"=w270) -> ("Colour Table"=w271:u32[])  [unwired: 10 in]
                  n159 = property on="B-Scan Chart" class="IntGraph (strict)"("Color Table"=w271) -> ()  [unwired: 2 in, 2 out]
                  n160 = property on="B-Scan Chart 2" class="IntGraph (strict)"("Color Table"=w271) -> ()  [unwired: 2 in, 2 out]
                }
                event "QUIT": Value Change {
                  # "set flag to stop acquisition loop"
                  n161 = event-data() -> ()  [unwired: 1 in, 6 out]
                  "Stop" <- TRUE ("Stop")
                }
              }
            }
            n162 = while {
              tunnel: [w97] -> w63
              shift-right: [w95] -> w60
              shift-left: w65 -> [w93]
              shift-right: [w94] -> w64
              shift-left: w65 -> [w92]
              stop <- w96 stop-if-true
              # "Asynchronous Read from Micropulse"
              n163 = call <instrlib>:"Read MP Message.vi"() -> ("error out"=w91:errorcluster, "scan data info"=w98:T37, "Instrument Message"=w101:string)  [unwired: 7 in, 2 out]
              n164 = call <instrlib>:"Instrument Message History.vi"("Instrument Message"=w101) -> ("Message History out"=→"System Messages":string)  [unwired: 9 in, 1 out]
              n165 = Unbundle By Name(w98) -> ("Test No."=w99:u32)
              n166 = Unbundle By Name(w91) -> ("code"=w90:i32)
              n167 = case shown="0, Default" w90 {
                tunnel: w99 -> [w109 _]
                tunnel: w98 -> [w108 _]
                tunnel: [w107 w158] -> w97
                tunnel: [w106 w156] -> w95
                tunnel: [w105 w157] -> w94
                tunnel: w93 -> [w104 w156]
                tunnel: w92 -> [w103 w157]
                tunnel: w91 -> [w102 w158]
                frame 0, Default {
                  n168 = case shown="2" w109 {
                    selector: w109 -> [_ w113 w139]
                    tunnel: w108 -> [_ w114 w143]
                    tunnel: w102 -> [w112 w124 w148]
                    tunnel: [w112 w122 w145] -> w107
                    tunnel: [w110 w116 w134] -> w106
                    tunnel: [w111 w118 w133] -> w105
                    tunnel: w104 -> [w110 w117 _]
                    tunnel: w103 -> [w111 _ w140]
                    frame -1, Default {
                    }
                    frame 1 {
                      # "These helper VIs maintain internal information for each test.\nYou should use a different instance of these VIs for each test."
                      n169 = local read "Timed Scan definition"() -> (w121:T20)
                      n170 = call <instrlib>:"AScan+Peaks to XY Chart.vi"("error in (no error)"=w124, "scan data info"=w114, "Test No."=w113) -> ("error out"=w122:errorcluster, "AScan+Peaks"=→"A-Scan + Peaks":cluster{"timebase":dbl[], "data":u16[]}[], "Running Average PRF"=→"running average PRF":dbl)  [unwired: 3 in, 3 out]
                      "live error out" <- w122
                      n171 = call <instrlib>:"B-Scan (Timed) DVR - MultiChannel.vi"("Scan definition"=w121, "scan data info"=w114, "Test #"=w113) -> ("Update Display?"=w115:bool, "data value reference"=w119:refnum<data-value>)  [unwired: 4 in, 3 out]
                      n172 = case shown="True" w115 {
                        tunnel: w119 -> [w126 w130]
                        tunnel: [w126 w128] -> w118
                        tunnel: w117 -> [w125 w127]
                        tunnel: [w125 w127] -> w116
                        frame False {
                        }
                        frame True {
                          n173 = in-place {
                            in-place-border: [w131] -> w129
                            n174 = in-place-dvr #1(w130) -> (w131:u16[][])  [unwired: 1 out]
                            n175 = in-place-dvr #1(w131) -> (w128:refnum<data-value>)  [unwired: 1 out]
                          }
                          "B-Scan Chart" <- w129
                        }
                      }
                    }
                    frame 2 {
                      n176 = local read "Timed Scan definition"() -> (w141:T20)
                      n177 = call <instrlib>:"AScan+Peaks to XY Chart.vi"("error in (no error)"=w148, "scan data info"=w143, "Test No."=w139) -> ("error out"=w145:errorcluster, "AScan+Peaks"=→"A-Scan + Peaks 2":cluster{"timebase":dbl[], "data":u16[]}[], "Running Average PRF"=→"running average PRF 2":dbl)  [unwired: 3 in, 3 out]
                      "live error out 2" <- w145
                      n178 = call <instrlib>:"B-Scan (Timed) DVR - MultiChannel.vi"("Scan definition"=w141, "scan data info"=w143, "Test #"=w139) -> ("Update Display?"=w142:bool, "B-Scan In Progress?"=→"B-Scan In Progress?":bool, "B-Scan Finished?"=w135:bool, "data value reference"=w144:refnum<data-value>)  [unwired: 4 in, 1 out]
                      n179 = case shown="True" w142 {
                        tunnel: w144 -> [w150 w154]
                        tunnel: [w150 w152] -> w137
                        tunnel: [w149 w151] -> w136
                        tunnel: w140 -> [w149 w151]
                        frame False {
                        }
                        frame True {
                          n180 = in-place {
                            in-place-border: [w155] -> w153
                            n181 = in-place-dvr #2(w154) -> (w155:u16[][])  [unwired: 1 out]
                            n182 = in-place-dvr #2(w155) -> (w152:refnum<data-value>)  [unwired: 1 out]
                          }
                          "B-Scan Chart 2" <- w153
                        }
                      }
                      n183 = call <instrlib>:"06-5-Save B-Scans To Disk.vi"("Enable Logging?"="Log Data?", "DVR Test 2"=w137, "DVR Test 1"=w136, "B-Scan Finished?"=w135) -> ("DVR Test 2 out"=w134:refnum<data-value>, "DVR Test 1 out"=w133:refnum<data-value>)  [unwired: 6 in]
                    }
                  }
                }
                frame 56 {
                  # "Error code is 56 - timeout error - no data coming from MicroPulse"
                }
              }
              n184 = flat-sequence {
                tunnel: [w159] -> w96
                tunnel: w97 -> [_]
                frame #0 {
                  n185 = local read "Stop"() -> (w159:bool)
                }
              }
            }
            n186 = Delete Data Value Reference(data value reference=w64, error in=w63) -> (error out=w62:errorcluster)  [unwired: 1 out]
            n187 = Delete Data Value Reference(data value reference=w60, error in=w62) -> (error out=w61:errorcluster)  [unwired: 1 out]
          }
          frame Error {
          }
        }
        n188 = Select(t=Main_Program_State_-_Enum."Reset HW", s=w55, f=Main_Program_State_-_Enum."Shutdown") -> (s? t:f=w54:T23)
      }
      frame "Reset HW" {
        # "Close the connection to allow for reopening in the \"Init HW\" case"
        n189 = call <instrlib>:"Close.vi"("error in (no error)"=w276) -> ("error out"=w275:errorcluster)  [unwired: 9 in, 1 out]
      }
      frame "Shutdown" {
        # "Terminate the TCP/IP connection"
        n190 = local write "Stop"(FALSE ("stop")) -> ()
        n191 = call <instrlib>:"Close.vi"() -> ()  [unwired: 10 in, 2 out]
      }
    }
  }
